vi "Update Parent (String).vi"(8 "error in (no error)":errorcluster, 10 "Parent Name":string, 11 "ControlClassWizard in":refnum<class "QControl Creation Wizard.lvclass">) -> (0 "error out":errorcluster, 3 "ControlClassWizard (dup)":refnum<class "QControl Creation Wizard.lvclass">)   [LabVIEW 2023, in "QControl Creation Wizard.lvclass"]
doc: "<b> </b> <b> </b>\n©2016 Q Software Innovations, LLC (QSI)\nwritten by Quentin Alldredge\nproduced in LabVIEW 2015\n\nsupport@qsoftwareinnovations.com\nwww.qsoftwareinnovations.com\n\nAll rights reserved.\n\nRedistribution and use in source and binary forms, with or without modification, are permitted provided that the following conditions are met:\n\n * Redistributions of source code must retain the above copyright notice, this list of conditions and the following disclaimer.\n * Redistributions in binary form must reproduce the above copyright notice, this list of conditions and the following disclaimer in the documentation and/or other materials provided with the distribution.\n * Neither the name of Q Software Innovations, LLC. nor the names of its contributors may be used to endorse or promote products derived from this software without specific prior written permission.\n\nTHIS SOFTWARE IS PROVIDED BY THE COPYRIGHT HOLDERS AND CONTRIBUTORS \"AS IS\" AND ANY EXPRESS OR IMPLIED WARRANTIES, INCLUDING, BUT NOT LIMITED TO, THE IMPLIED WARRANTIES OF MERCHANTABILITY AND FITNESS FOR A PARTICULAR PURPOSE ARE DISCLAIMED. IN NO EVENT SHALL THE COPYRIGHT OWNER OR CONTRIBUTORS BE LIABLE FOR ANY DIRECT, INDIRECT, INCIDENTAL, SPECIAL, EXEMPLARY, OR CONSEQUENTIAL DAMAGES (INCLUDING, BUT NOT LIMITED TO, PROCUREMENT OF SUBSTITUTE GOODS OR SERVICES; LOSS OF USE, DATA, OR PROFITS; OR BUSINESS INTERRUPTION) HOWEVER CAUSED AND ON ANY THEORY OF LIABILITY, WHETHER IN CONTRACT, STRICT LIABILITY, OR TORT (INCLUDING NEGLIGENCE OR OTHERWISE) ARISING IN ANY WAY OUT OF THE USE OF THIS SOFTWARE, EVEN IF ADVISED OF THE POSSIBILITY OF SUCH DAMAGE."
uses:
  QControl Creation Wizard.lvclass
  QControl Creation Wizard.lvclass/QControl Creation Wizard.ctl
  New QControl Info/New QControl Info.lvclass/New QControl Info.ctl
  New QControl Info/Write Parent Class Path.vi
  <vilib>/Utility/error.llb/Error Cluster From Error Code.vi
  <vilib>/ErrorRing/Error Ring.xnode
  New QControl Info/New QControl Info.lvclass
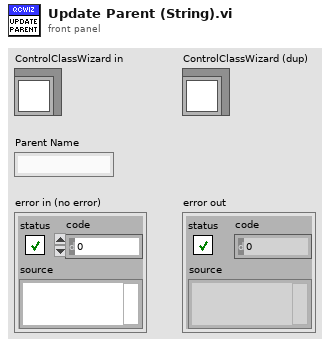
[diagram p1: front panel]
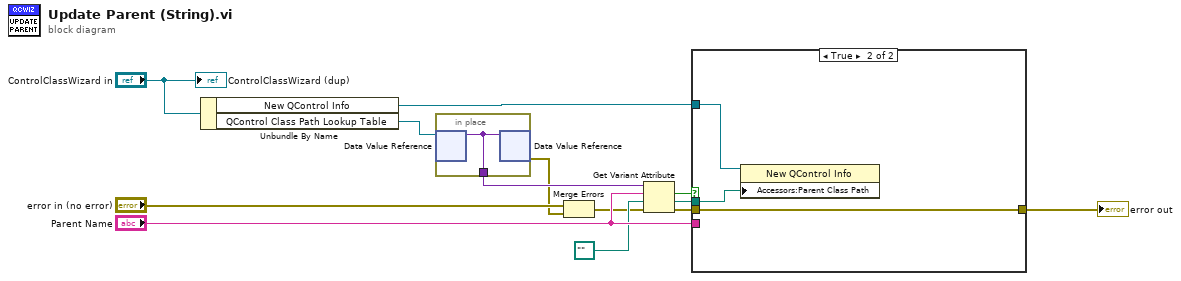
[diagram p0: block diagram]
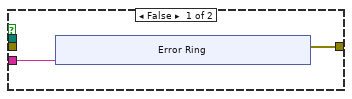
[diagram p2: hidden frame]
diagram:
  n1 = Unbundle By Name("ControlClassWizard in") -> ("New QControl Info"=w6:refnum<data-value>, "QControl Class Path Lookup Table"=w4:refnum<data-value>)
  n2 = in-place {
    in-place-border: [w14] -> w3
    n3 = in-place-dvr #1(w4) -> (w14:variant)  [unwired: 1 out]
    n4 = in-place-dvr #1(w14) -> (w1:errorcluster)  [unwired: 1 out]
  }
  n5 = Merge Errors("error in (no error)", w1) -> (w2:errorcluster)
  n6 = Get Variant Attribute(Variant=w3, name="Parent Name", default value (empty Variant)=path "", error in=w2) -> (found=w8:bool, value=w9:path, error out=w7:errorcluster)  [unwired: 1 out]
  n7 = case shown="True" w8 {
    tunnel: w9 -> [_ w24]
    tunnel: w7 -> [_ w26]
    tunnel: [w15 w26] -> w12
    tunnel: "Parent Name" -> [w16 _]
    tunnel: w6 -> [_ w25]
    frame False {
      n8 = xnode "Error Ring"("parameter 0"=w16) -> ("error out"=w15:errorcluster)
    }
    frame True {
      n9 = property class="New QControl Info"(reference=w25, "Accessors:Parent Class Path"=w24) -> ()  [unwired: 1 in, 2 out]
    }
  }
  "error out" <- w12
  "ControlClassWizard (dup)" <- "ControlClassWizard in"
